vi "TDC_getDeviceInfo.vi"(8 "Error In":errorcluster, 11 "Device Number":i32) -> (0 "Error Out":errorcluster, 1 "Connected":bool, 2 "Serial Number":string, 3 "Device ID":i32, 5 "Device Type":u16(ring) items=["quTAG", "No Device"])   [LabVIEW 2011]
uses:
  tdcbase.dll
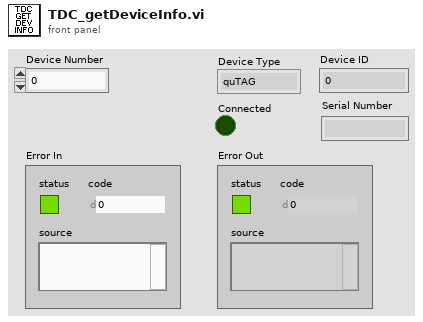
[diagram p1: front panel]
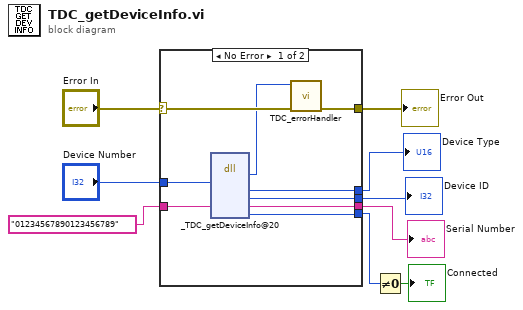
[diagram p0: block diagram]
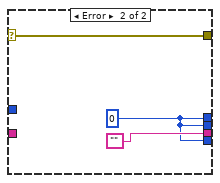
[diagram p2: hidden frame]
diagram:
  n1 = case shown="No Error" "Error In" {
    selector: "Error In" -> [w18 w21]
    tunnel: [w17 w21] -> w8
    tunnel: "Device Number" -> [w15 _]
    tunnel: [w14 w19] -> w1
    tunnel: [w13 w19] -> w2
    tunnel: [w12 ""] -> w3
    tunnel: [w11 w19] -> w4
    tunnel: "01234567890123456789" -> [w10 _]
    frame No Error {
      n2 = dll-call lib="X:/tdcbase.dll" fn="_TDC_getDeviceInfo@20"("devNo"=w15, "serialNo"=w10) -> ("return type"=w16:i32, "devType"=w14:i32, "devId"=w13:i32, "serialNo"=w12:string, "connected"=w11:i32)  [unwired: 7 in, 2 out]
      n3 = call "TDC_errorHandler.vi"("Error In"=w18, "TDC Return Code"=w16) -> ("Error Out"=w17:errorcluster)  [unwired: 9 in]
    }
    frame Error {
      w19 = 0
    }
  }
  "Error Out" <- w8
  "Device ID" <- w2
  "Serial Number" <- w3
  "Device Type" <- w1
  n4 = Not Equal To 0?(x=w4) -> (x != 0?=→"Connected":bool)
